vi "checkin.vi"(8 "error in (no error)":errorcluster, 11 "GenericDataCollection in":refnum<class "GenericDataCollection.lvclass">) -> (0 "error out":errorcluster, 3 "GenericDataCollection out":refnum<class "GenericDataCollection.lvclass">)   [LabVIEW 2010, in "GenericDataCollection.lvclass"]
uses:
  GenericDataCollection.lvclass
  common/classes/GenericToplevelComponent/GenericToplevelComponent/GenericToplevelComponent.lvclass
  class_data.vi
  common/classes/GenericComponent/GenericComponent/GenericComponent.lvclass
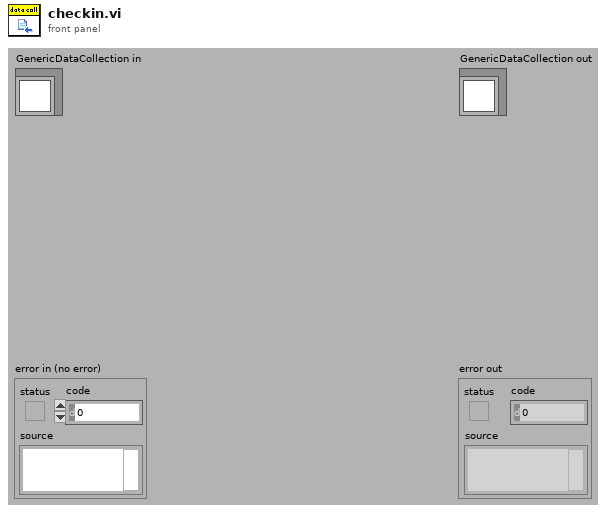
[diagram p1: front panel]
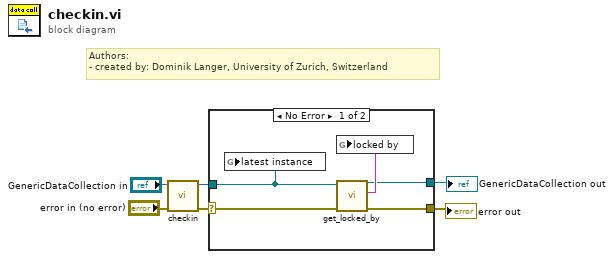
[diagram p0: block diagram]
diagram:
  # "Authors: \n- created by: Dominik Langer, University of Zurich, Switzerland"
  n1 = call-parent "checkin.vi"("error in (no error)"="error in (no error)", "GenericPlugin in"="GenericDataCollection in") -> ("error out"=w3:errorcluster, "GenericPlugin out"=w1:refnum<class "GenericDataCollection.lvclass">)  [unwired: 8 in]
  n2 = case shown="No Error" w3 {
    selector: w3 -> [w8 w13]
    tunnel: [w10 w13] -> w5
    tunnel: [w9 w12] -> w6
    tunnel: w1 -> [w7 w12]
    frame No Error {
      n3 = global write "class_data.vi" "latest instance"(w7) -> ()
      n4 = call "get_locked_by.vi"("error in (no error)"=w8, "GenericPlugin.lvclass in"=w7) -> ("error out"=w10:errorcluster, "locked by"=w11:string, "GenericPlugin.lvclass out"=w9:refnum<class "GenericDataCollection.lvclass">)  [unwired: 7 out]
      n5 = global write "class_data.vi" "locked by"(w11) -> ()
    }
    frame Error {
    }
  }
  "error out" <- w5
  "GenericDataCollection out" <- w6
